vi "Parse.vi"(7 "channel blocks":T1[](array[typedef]) {"buffer offset" format="%d bytes"}, 8 "error in (no error)":errorcluster, 9 "dst Buffer":refnum<class "DBL Pointer.lvclass">, 10 "src Buffer":refnum<class "Buffer.lvclass">, 11 "Buffer Converter in":refnum<class "Buffer Converter.lvclass">) -> (0 "error out":errorcluster, 3 "Buffer Converter out":refnum<class "Buffer Converter.lvclass">)   [LabVIEW 2017, in "DSF Core.lvlib" / "Buffer Converter.lvclass"]
uses:
  Buffer Converter.lvclass
  Pointer/DBL Pointer.lvclass
  Buffer/Buffer.lvclass
  Configuration/Public/Controls/DSF Engine Channel Configuration.ctl
  Configuration/Public/Controls/DSF Data Type.ctl
  Buffer Converter.lvclass/Buffer Converter.ctl
  DSF Core.lvlib
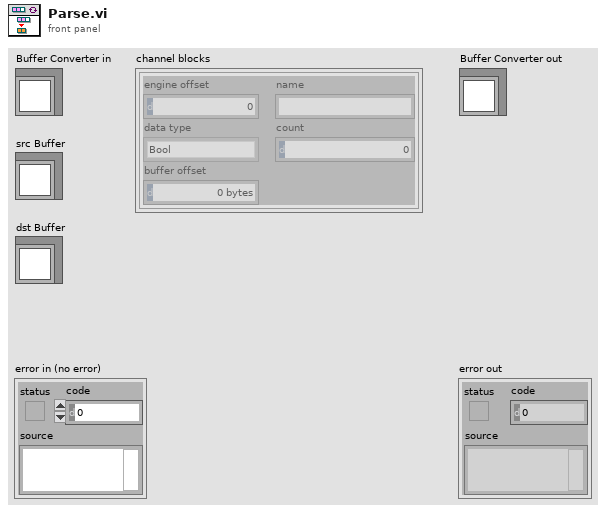
[diagram p1: front panel]
types:
  T1 = typedef "DSF Core.lvlib/DSF Engine Channel Configuration.ctl" = cluster{"engine offset":u64, "name":string, "data type":T2, "count":u64, "buffer offset":u64}
  T2 = typedef "DSF Core.lvlib/DSF Data Type.ctl" = enum8{"Bool", "SGL", "DBL", "I8", "I16", "I32", "I64", "U8", "U16", "U32", "U64"}
  T3 = typedef "DSF Core.lvlib/DSF Runtime Type Buffers.ctl" = cluster{"Bool":bool[], "SGL":sgl[], "DBL":dbl[], "I8":i8[], "I16":i16[], "I32":i32[], "I64":i64[], "U8":u8[], "U16":u16[], "U32":u32[], "U64":u64[]}
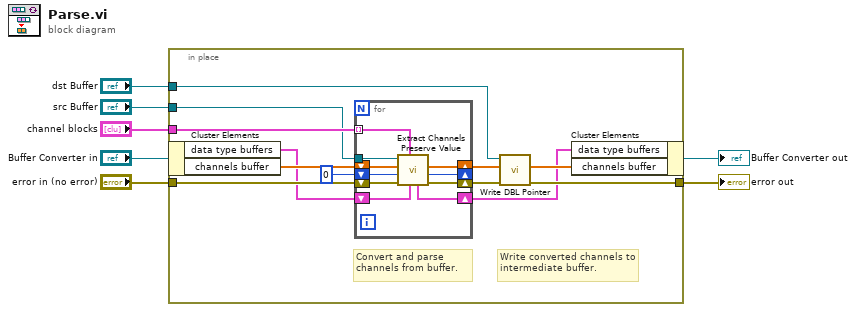
[diagram p0: block diagram]
diagram:
  n1 = in-place {
    in-place-border: "channel blocks" -> [w13]
    in-place-border: "dst Buffer" -> [w12]
    in-place-border: "error in (no error)" -> [w14]
    in-place-border: "src Buffer" -> [w11]
    in-place-border: [w10] -> w1
    # "Write converted channels to intermediate buffer."
    # "Convert and parse channels from buffer."
    n2 = in-place-cluster #1("Buffer Converter in") -> ("data type buffers"=w9:T3, "channels buffer"=w15:dbl[])
    n3 = for {
      shift-right: [w28] -> w19
      shift-left: w15 -> [w26]
      shift-right: [w29] -> w18
      shift-left: w14 -> [w27]
      tunnel: w11 -> [w25]
      tunnel: w13 -> [w22] mode=indexing
      shift-right: [w24] -> w8
      shift-left: w9 -> [w23]
      shift-right: [w21] -> _
      shift-left: u64 0 ("channels buffer index in") -> [w20]
      n4 = call "Extract Channels Preserve Value.vi"("data type buffers in"=w23, "channel block"=w22, "error in (no error)"=w27, "channels buffer index in"=w20, "channels buffer in"=w26, "Buffer in"=w25) -> ("error out"=w29:errorcluster, "channels buffer index out"=w21:u64, "channels buffer out"=w28:dbl[], "data type buffers out"=w24:T3)  [unwired: 1 in, 1 out]
    }
    n5 = call "Write DBL Pointer.vi"("error in (no error)"=w18, "buffer in"=w19, "DBL Pointer in"=w12) -> ("error out"=w10:errorcluster, "buffer out"=w16:dbl[])  [unwired: 6 in, 1 out]
    n6 = in-place-cluster #1("data type buffers"=w8, "channels buffer"=w16) -> (→"Buffer Converter out":refnum<class "Buffer Converter.lvclass">)
  }
  "error out" <- w1
